vi "2 LED Serial Sequence With ForLoop.vi"(5 "Completed Tag name":string="Boolean processing result 0", 6 "Jump Tag Name":string="Boolean processing result 0", 7 "Iteration Tag Name":string="Boolean processing result 0", 8 "Tag Name 2":string="Boolean processing result 0", 9 "Tag Name 1":string="Boolean processing result 0", 10 "Name":string="Led Sequence") -> (2 "Sequence out":refnum<class "Sequence Config.lvclass">)   [LabVIEW 2015, in "Sequencer Module tests.lvlib"]
uses:
  Sequencer Module tests.lvlib
  classes/Sequence/Config/Sequence Config.lvclass
  basic steps/Wait Step/Config/Wait Step Config.lvclass
  <vilib>/NI/Tag Bus Module Framework/channel/channel classification.ctl
  <vilib>/NI/Tag Bus/tag/Data Type.ctl
  basic steps/Conditional Jump Step/Config/Conditional Jump Step Config.lvclass
  basic steps/Counter/Config/Counter Config.lvclass
  basic steps/Update Tag Step/Config/Update Tag Configuration/Update Tag Config.lvclass
  <vilib>/NI/Tag Bus/tag/tag descriptor.lvclass/tag descriptor.ctl
  <vilib>/NI/Tag Bus/tag/tag descriptor.lvclass
  <vilib>/NI/Tag Bus Module Framework/channel/TBM channel.lvclass
panel:
  out "Array":string[](array[string])
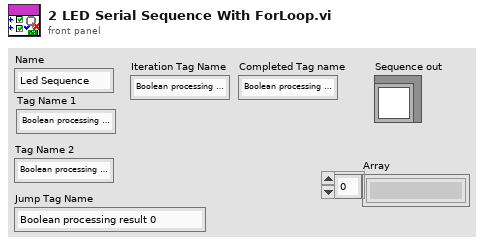
[diagram p1: front panel]
types:
  T1 = typedef "TBM channel.lvclass/channel classification.ctl" = enum16{"input data", "output data", "processing parameter", "processing result"}
  T2 = typedef "tag bus.lvlib/tag descriptor.lvclass/Data Type.ctl" = enum16{"Double", "Single", "I64", "I32", "I16", "I8", "U64", "U32", "U16", "U8", "Boolean", "String", "Array of Double", "Array of Single", "Array of I64", "Array of I32", "Array of I16", "Array of I8", "Array of U64", "Array of U32", "Array of U16", "Array of U8", "Array of Boolean", "Array of String"}
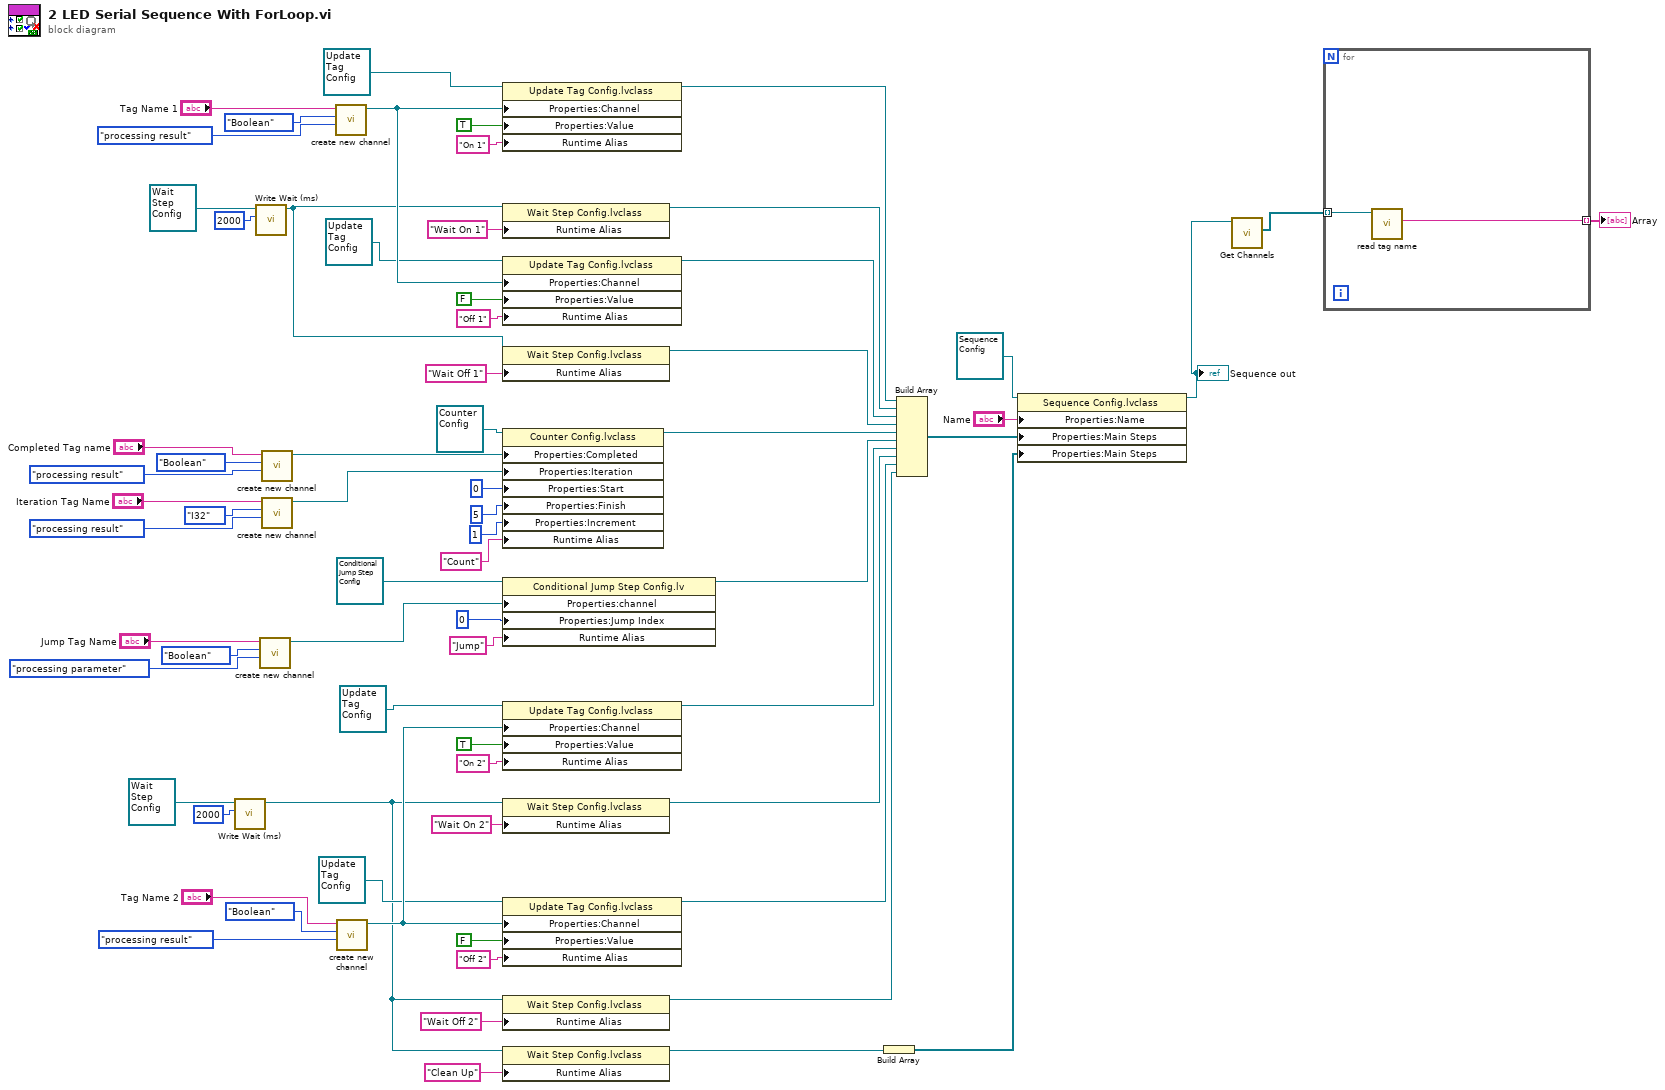
[diagram p0: block diagram]
diagram:
  n1 = call-dynamic "Write Wait (ms).vi"("Wait (ms)"=u32 2000, "Wait Step in"=refnum<class "Wait Step Config.lvclass"> refnum ("Wait Step Config.lvclass")) -> ("Wait Step out"=w4:refnum<class "Wait Step Config.lvclass">)  [unwired: 8 in, 1 out]
  n2 = call-dynamic "Write Wait (ms).vi"("Wait (ms)"=u32 2000, "Wait Step in"=refnum<class "Wait Step Config.lvclass"> refnum ("Wait Step Config.lvclass")) -> ("Wait Step out"=w18:refnum<class "Wait Step Config.lvclass">)  [unwired: 8 in, 1 out]
  n3 = call <vilib>:"create new channel.vi"("channel classification"=channel_classification."processing parameter", "data type"=Data_Type."Boolean" ("Data Type"), "channel name"="Jump Tag Name") -> ("channel"=w39:refnum<class "TBM channel.lvclass">)  [unwired: 8 in]
  n4 = call <vilib>:"create new channel.vi"("channel classification"=channel_classification."processing result", "data type"=Data_Type."Boolean" ("Data Type"), "channel name"="Completed Tag name") -> ("channel"=w36:refnum<class "TBM channel.lvclass">)  [unwired: 8 in]
  n5 = call <vilib>:"create new channel.vi"("channel classification"=channel_classification."processing result", "data type"=Data_Type."I32" ("Data Type"), "channel name"="Iteration Tag Name") -> ("channel"=w40:refnum<class "TBM channel.lvclass">)  [unwired: 8 in]
  n6 = call <vilib>:"create new channel.vi"("channel classification"=channel_classification."processing result", "data type"=Data_Type."Boolean" ("Data Type"), "channel name"="Tag Name 1") -> ("channel"=w61:refnum<class "TBM channel.lvclass">)  [unwired: 8 in]
  n7 = call <vilib>:"create new channel.vi"("channel classification"=channel_classification."processing result", "data type"=Data_Type."Boolean" ("Data Type"), "channel name"="Tag Name 2") -> ("channel"=w57:refnum<class "TBM channel.lvclass">)  [unwired: 8 in]
  n8 = property class="Update Tag Config.lvclass"(reference=refnum<class "Update Tag Config.lvclass"> refnum ("Update Tag Config.lvclass"), "Properties:Channel"=w61, "Properties:Value"=TRUE, "Runtime Alias"="On 1") -> (reference out=w48:refnum<class "Update Tag Config.lvclass">)  [unwired: 1 in, 1 out]
  n9 = property class="Wait Step Config.lvclass"(reference=w18, "Runtime Alias"="Wait On 1") -> (reference out=w24:refnum<class "Wait Step Config.lvclass">)  [unwired: 1 in, 1 out]
  n10 = property class="Update Tag Config.lvclass"(reference=refnum<class "Update Tag Config.lvclass"> refnum ("Update Tag Config.lvclass"), "Properties:Channel"=w61, "Properties:Value"=FALSE, "Runtime Alias"="Off 1") -> (reference out=w47:refnum<class "Update Tag Config.lvclass">)  [unwired: 1 in, 1 out]
  n11 = property class="Wait Step Config.lvclass"(reference=w18, "Runtime Alias"="Wait Off 1") -> (reference out=w23:refnum<class "Wait Step Config.lvclass">)  [unwired: 1 in, 1 out]
  n12 = property class="Counter Config.lvclass"(reference=refnum<class "Counter Config.lvclass"> refnum ("Counter Config.lvclass"), "Properties:Completed"=w36, "Properties:Iteration"=w40, "Properties:Start"=0 ("Start"), "Properties:Finish"=5 ("Finish"), "Properties:Increment"=1 ("Increment"), "Runtime Alias"="Count") -> (reference out=w35:refnum<class "Counter Config.lvclass">)  [unwired: 1 in, 1 out]
  n13 = property class="Conditional Jump Step Config.lv"(reference=refnum<class "Conditional Jump Step Config.lvclass"> refnum ("Conditional Jump Step Config.lvclass"), "Properties:channel"=w39, "Properties:Jump Index"=0 ("Jump Index"), "Runtime Alias"="Jump") -> (reference out=w14:refnum<class "Conditional Jump Step Config.lvclass">)  [unwired: 1 in, 1 out]
  n14 = property class="Update Tag Config.lvclass"(reference=refnum<class "Update Tag Config.lvclass"> refnum ("Update Tag Config.lvclass"), "Properties:Channel"=w57, "Properties:Value"=TRUE, "Runtime Alias"="On 2") -> (reference out=w13:refnum<class "Update Tag Config.lvclass">)  [unwired: 1 in, 1 out]
  n15 = property class="Wait Step Config.lvclass"(reference=w4, "Runtime Alias"="Wait On 2") -> (reference out=w12:refnum<class "Wait Step Config.lvclass">)  [unwired: 1 in, 1 out]
  n16 = property class="Update Tag Config.lvclass"(reference=refnum<class "Update Tag Config.lvclass"> refnum ("Update Tag Config.lvclass"), "Properties:Channel"=w57, "Properties:Value"=FALSE, "Runtime Alias"="Off 2") -> (reference out=w11:refnum<class "Update Tag Config.lvclass">)  [unwired: 1 in, 1 out]
  n17 = property class="Wait Step Config.lvclass"(reference=w4, "Runtime Alias"="Wait Off 2") -> (reference out=w10:refnum<class "Wait Step Config.lvclass">)  [unwired: 1 in, 1 out]
  n18 = property class="Wait Step Config.lvclass"(reference=w4, "Runtime Alias"="Clean Up") -> (reference out=w16:refnum<class "Wait Step Config.lvclass">)  [unwired: 1 in, 1 out]
  n19 = Build Array(w16) -> (w15:refnum<class "Wait Step Config.lvclass">[])
  n20 = Build Array(w48, w24, w47, w23, w35, w14, w13, w12, w11, w10) -> (w69:refnum<class "Step Config.lvclass">[])
  n21 = property class="Sequence Config.lvclass"(reference=refnum<class "Sequence Config.lvclass"> refnum ("Sequence Config.lvclass"), "Properties:Name"="Name", "Properties:Main Steps"=w69, "Properties:Main Steps"=w15) -> (reference out=w3:refnum<class "Sequence Config.lvclass">)  [unwired: 1 in, 1 out]
  "Sequence out" <- w3
  n22 = call "Get Channels.vi"("Sequence Config in"=w3) -> ("Channels"=w2:refnum<class "TBM channel.lvclass">[])  [unwired: 8 in, 2 out]
  n23 = for {
    tunnel: w2 -> [w71] mode=indexing
    tunnel: [w70] -> w1 mode=indexing
    n24 = call <vilib>:"read tag name.vi"("system tag in"=w71) -> ("name"=w70:string)  [unwired: 8 in, 2 out]
  }
  "Array" <- w1
